vi "RichToFlatnise_SessionInformation.vi"(5 "OutputClusterType":T1, 11 "InputCluster":T2) -> (3 "OutputCluster":T1)   [LabVIEW 2021, in "basic_switch_executive_driver_client.lvlib"]
uses:
  basic_switch_executive_driver_client.lvlib
  nise_SessionInformation.ctl
  <vilib>/Plug-In SDKs/Clients/Session Management V1/Session Reservation/Initialize and Close Session Behavior.ctl
  nise_SessionInformation_Flat.ctl
  <vilib>/Plug-In SDKs/Clients/Session Management V1/Session Reservation/Session Reservation.lvclass
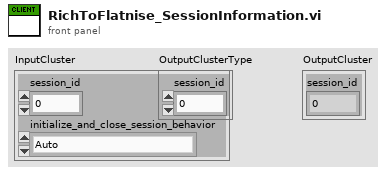
[diagram p1: front panel]
types:
  T1 = typedef "basic_switch_executive_driver_client.lvlib/nise_SessionInformation_Flat.ctl" = cluster{"session_id":u32}
  T2 = typedef "basic_switch_executive_driver_client.lvlib/nise_SessionInformation.ctl" = cluster{"session_id":u32, "initialize_and_close_session_behavior":T3}
  T3 = typedef "NI Session Management V1 Client.lvlib/Session Reservation.lvclass/Initialize and Close Session Behavior.ctl" = enum16{"Auto", "Initialize and Close", "Attach and Detach", "Initialize and Detach", "Attach and Close"}
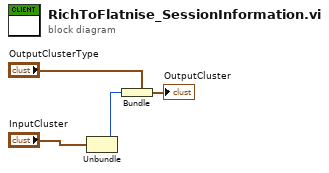
[diagram p0: block diagram]
diagram:
  n1 = Unbundle "Unbundle"("InputCluster") -> ("session_id"=w1:u32)  [unwired: 1 out]
  n2 = Bundle "Bundle"(cluster="OutputClusterType", "session_id"=w1) -> (→"OutputCluster":T1)
